vi "Pololu.Mgr - Store Stop Position.vi"(6 "Type":enum16{"Lower", "Upper"}(ring), 8 "error in (no error)":errorcluster, 9 "Pos(Deg)":dbl, 10 "Channel":u8, 11 "PololuCtrl in":refnum<class "PololuCtrl.lvclass">) -> (0 "error out":errorcluster, 3 "PololuCtrl out":refnum<class "PololuCtrl.lvclass">)   [LabVIEW 2018, in "PololuCtrl.lvclass"]
uses:
  PololuCtrl.lvclass
  PololuCtrl.lvclass/PololuCtrl.ctl
  SubVIs/Pololu.Message Byte Defs.ctl
  Serial Port/Class/SerialPort.lvclass
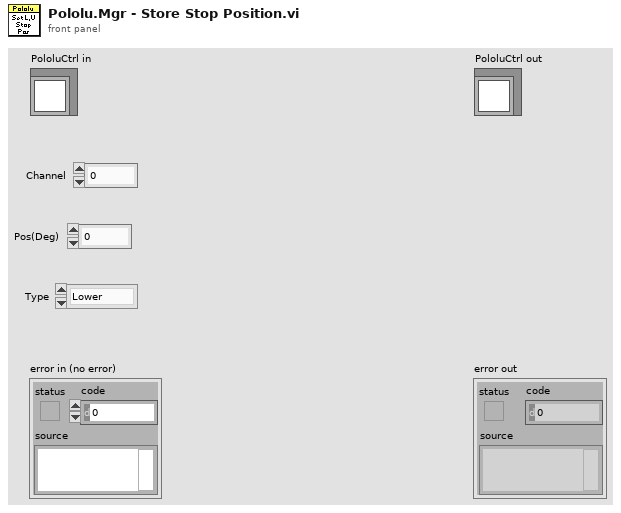
[diagram p1: front panel]
types:
  T1 = typedef "Pololu.Device Config.ctl" = cluster{"Chan":u8, "Accel":u16, "Speed":u16, "Positions":dbl[], "Range Info":T2}
  T2 = typedef "Pololu.Device Range Config.ctl" = cluster{"Min us":dbl, "Max us":dbl, "Min deg":dbl, "Max deg":dbl, "LStopDeg":dbl, "UStopDeg":dbl}
  T3 = cluster{"Channel":u8, "Pos":u16, "Response":u16, "Bytes":u8[], "Query":bool}
  T4 = typedef "Pololu.Message Byte Defs.ctl" = u8
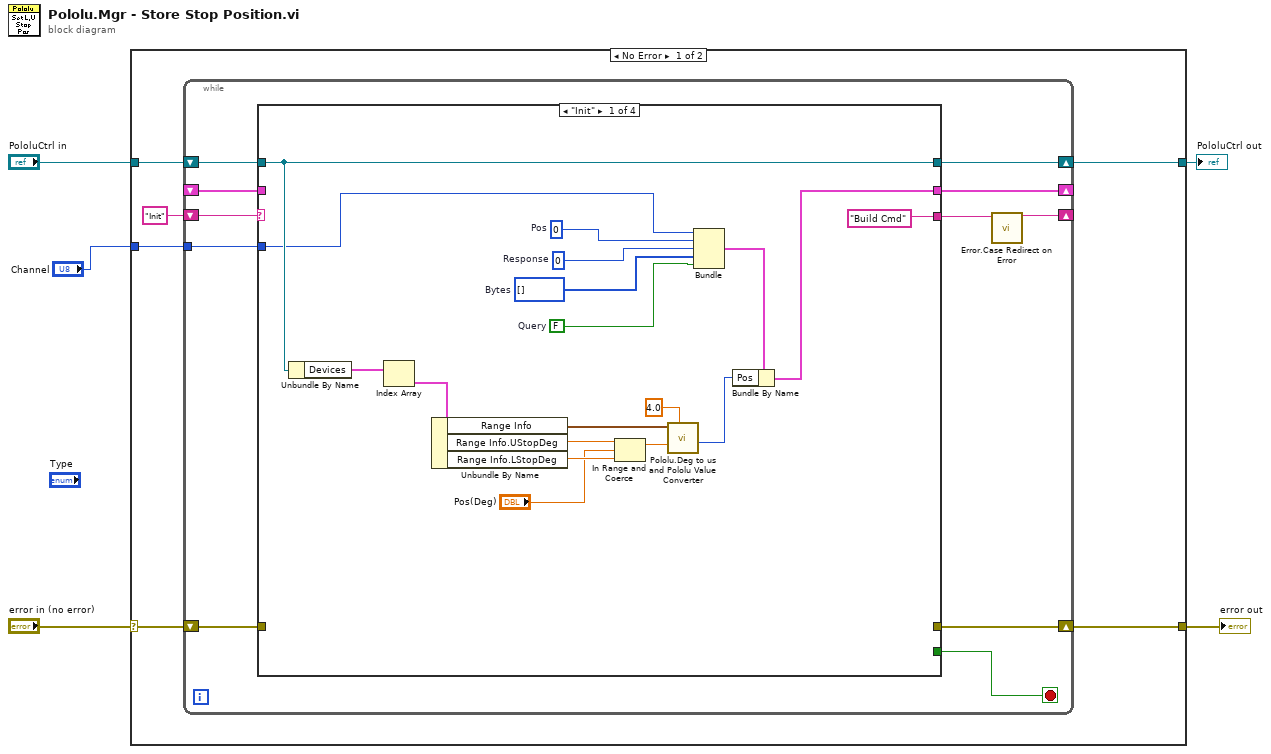
[diagram p0: block diagram]
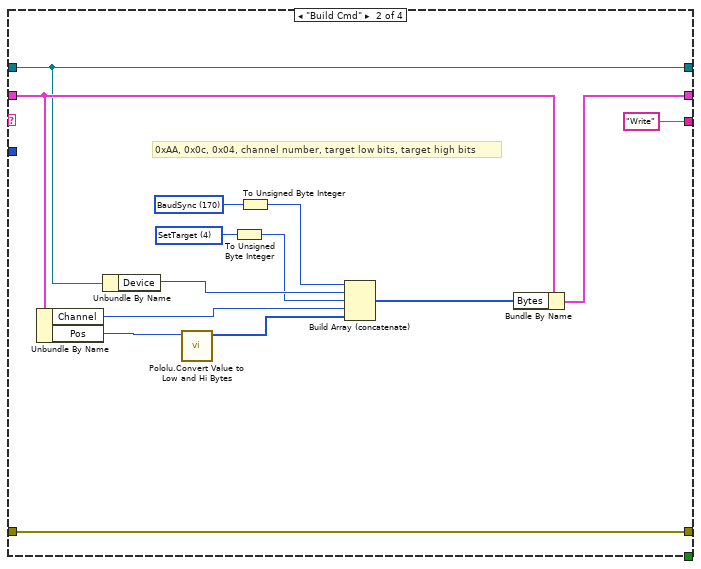
[diagram p2: hidden frame]
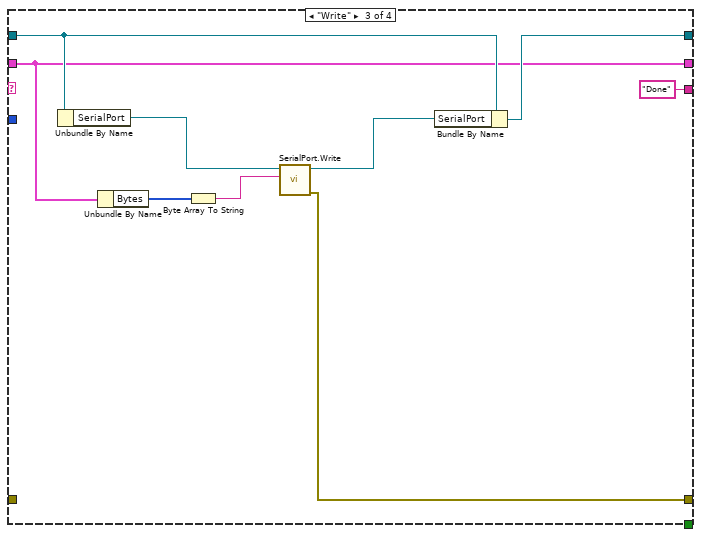
[diagram p3: hidden frame]
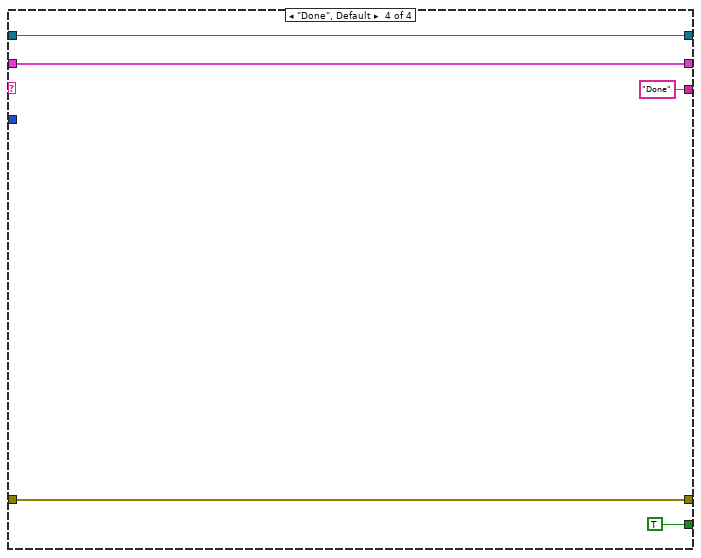
[diagram p4: hidden frame]
diagram:
  n1 = case shown="No Error" "error in (no error)" {
    selector: "error in (no error)" -> [w10 w70]
    tunnel: [w7 w70] -> w4
    tunnel: [w9 w69] -> w2
    tunnel: "PololuCtrl in" -> [w11 w69]
    tunnel: "Channel" -> [w6 _]
    frame No Error {
      n2 = while {
        shift-right: [w21] -> w9
        shift-left: w11 -> [w22]
        shift-right: [w14] -> w7
        shift-left: w10 -> [w15]
        shift-right: [w18] -> _
        shift-left: "Init" -> [w19]
        shift-right: [w16] -> _
        shift-left: _ -> [w20]
        tunnel: w6 -> [w12]
        stop <- w13 stop-if-true
        n3 = case shown="\"Init\"" w19 {
          tunnel: w22 -> [w35 w48 w60 w68]
          tunnel: [w35 w48 w61 w68] -> w21
          tunnel: w20 -> [_ w52 w56 w65]
          tunnel: ["Build Cmd" "Write" "Done" "Done"] -> w17
          tunnel: [w32 w53 w56 w65] -> w16
          tunnel: w15 -> [_ w54 _ w66]
          tunnel: [_ w54 w57 w66] -> w14
          tunnel: [_ _ _ TRUE] -> w13
          tunnel: w12 -> [w23 _ _ _]
          frame "Init" {
            w36 = u16 0  # Pos
            w39 = u16 0  # Response
            w37 = FALSE  # Query
            w38 = u8[] []  # Bytes
            n4 = Unbundle By Name(w35) -> ("Devices"=w34:T1[])
            n5 = Index Array(array=w34) -> (element=w31:T1)  [unwired: 1 in]
            n6 = Unbundle By Name(w31) -> ("Range Info"=w26:T2, "Range Info.UStopDeg"=w30:dbl, "Range Info.LStopDeg"=w29:dbl)
            n7 = In Range and Coerce(upper limit=w30, x="Pos(Deg)", lower limit=w29) -> (coerced(x)=w27:dbl)  [unwired: 1 out]
            n8 = call "Pololu.Deg to us and Pololu Value Converter.vi"("us to Units Mult"=4.0, "Set Pos (Deg)"=w27, "Range Info"=w26) -> ("Cmd units"=w25:u16)  [unwired: 7 in, 1 out]
            n9 = Bundle("Channel"=w23, "Pos"=w36, "Response"=w39, "Bytes"=w38, "Query"=w37) -> (w33:T3)  [unwired: 1 in]
            n10 = Bundle By Name(cluster=w33, "Pos"=w25) -> (w32:T3)
          }
          frame "Build Cmd" {
            w42 = T4 4 items=["BaudSync"=170, "SetTarget"=4, "Set Speed"=7, "Set Accel"=9, "Get Pos"=16, "Get MovStat"=19, "Get Errors"=33] ("Cmds")
            w43 = T4 170 items=["BaudSync"=170, "SetTarget"=4, "Set Speed"=7, "Set Accel"=9, "Get Pos"=16, "Get MovStat"=19, "Get Errors"=33] ("Cmds")
            # "0xAA, 0x0c, 0x04, channel number, target low bits, target high bits"
            n11 = Unbundle By Name(w52) -> ("Channel"=w51:u8, "Pos"=w50:u16)
            n12 = Unbundle By Name(w48) -> ("Device"=w47:u8)
            n13 = call "Pololu.Convert Value to Low and Hi Bytes.vi"("Value"=w50) -> ("Low_Hi Bytes"=w44:u8[])  [unwired: 10 in]
            n14 = To Unsigned Byte Integer(number=w42) -> (unsigned 8bit integer=w45:T4)
            n15 = To Unsigned Byte Integer(number=w43) -> (unsigned 8bit integer=w46:T4)
            n16 = Build Array (concatenate)(w46, w47, w45, w51, w44) -> (w49:T4[])
            n17 = Bundle By Name(cluster=w52, "Bytes"=w49) -> (w53:T3)
          }
          frame "Write" {
            n18 = Unbundle By Name(w60) -> ("SerialPort"=w59:refnum<class "SerialPort.lvclass">)
            n19 = Unbundle By Name(w56) -> ("Bytes"=w62:u8[])
            n20 = Byte Array To String(unsigned byte array=w62) -> (string=w55:string)
            n21 = call "SerialPort.Write.vi"("Data"=w55, "SerialPort in"=w59) -> ("error out"=w57:errorcluster, "SerialPort out"=w58:refnum<class "SerialPort.lvclass">)  [unwired: 6 in, 2 out]
            n22 = Bundle By Name(cluster=w60, "SerialPort"=w58) -> (w61:refnum<class "PololuCtrl.lvclass">)
          }
          frame "Done", Default {
          }
        }
        n23 = call "Error.Case Redirect on Error.vi"("Next Case"=w17) -> ("Next Case Out"=w18:string)  [unwired: 10 in]
      }
    }
    frame Error {
    }
  }
  "error out" <- w4
  "PololuCtrl out" <- w2
